vi "Stopping.vi"(7 "Actor in":refnum<class "Actor.lvclass">, 8 "Error in":errorcluster) -> (5 "Actor out":refnum<class "Actor.lvclass">)   [LabVIEW 2025, in "jettl.lvlib"]
uses:
  jettl.lvlib
  Actor/Actor.lvclass
  Teardown Location.ctl
  Stopped Msg/Tell Parent.vi
  Stopped Msg/Tell Child.vi
  Attributes/Attributes/Attributes.lvclass
  Transport/Transport/Transport.lvclass
  Stopped Msg/Stopped Msg.lvlib
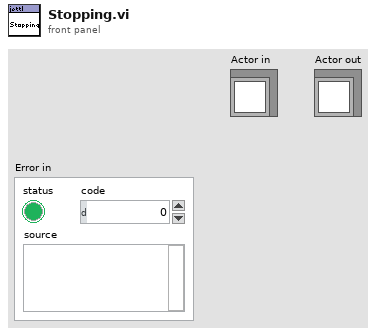
[diagram p1: front panel]
types:
  T1 = typedef "jettl.lvlib/Teardown Location.ctl" = enum16{"Start", "Stopping"}
  T2 = typedef "jettl.lvlib/Child UIDs.ctl" = set{string}
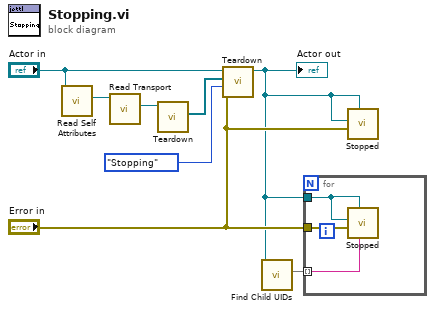
[diagram p0: block diagram]
diagram:
  n1 = call-dynamic "Read Self Attributes.vi"("Actor in"="Actor in") -> ("Self Attributes"=w5:refnum<class "Attributes.lvclass">)  [unwired: 10 in]
  n2 = call-dynamic "Read Transport.vi"("Attributes in"=w5) -> ("Transport"=w4:refnum<class "Transport.lvclass">)  [unwired: 10 in]
  n3 = call-dynamic "Teardown.vi"("Transport in"=w4) -> ("Unhandled Msgs"=w2:refnum<class "Msg.lvclass">[])  [unwired: 10 in]
  n4 = call-dynamic "Teardown.vi"("Error in"="Error in", "Teardown Location"=Teardown_Location."Stopping", "Unhandled Msgs"=w2, "Actor in"="Actor in") -> ("Actor out"=w6:refnum<class "Actor.lvclass">)  [unwired: 7 in]
  "Actor out" <- w6
  n5 = call-dynamic "Find Child UIDs.vi"("Actor in"=w6) -> ("Child UIDs"=w8:T2)  [unwired: 10 in]
  n6 = for {
    tunnel: w6 -> [w11]
    tunnel: w8 -> [w9] mode=indexing
    tunnel: "Error in" -> [w10]
    n7 = call-poly "Stopped.vi"("UID"=w9, "Actor in"=w11, "Error"=w10, "Actor"=w11) -> ()  [unwired: 7 in, 1 out]
  }
  n8 = call-poly "Stopped.vi"("Actor in"=w6, "Error"="Error in", "Actor"=w6) -> ()  [unwired: 8 in, 1 out]
